vi "set_Mode.vi"(6 "Array":T1(array[cluster]), 7 "Array 3":string[](array[string]), 10 "Array 2":T1(array[cluster])) -> (2 "settings needed":bool, 3 "spreadsheet string":string)   [LabVIEW 2013, in "Tapedrive_ESP301.lvclass"]
uses:
  Tapedrive_ESP301.lvclass
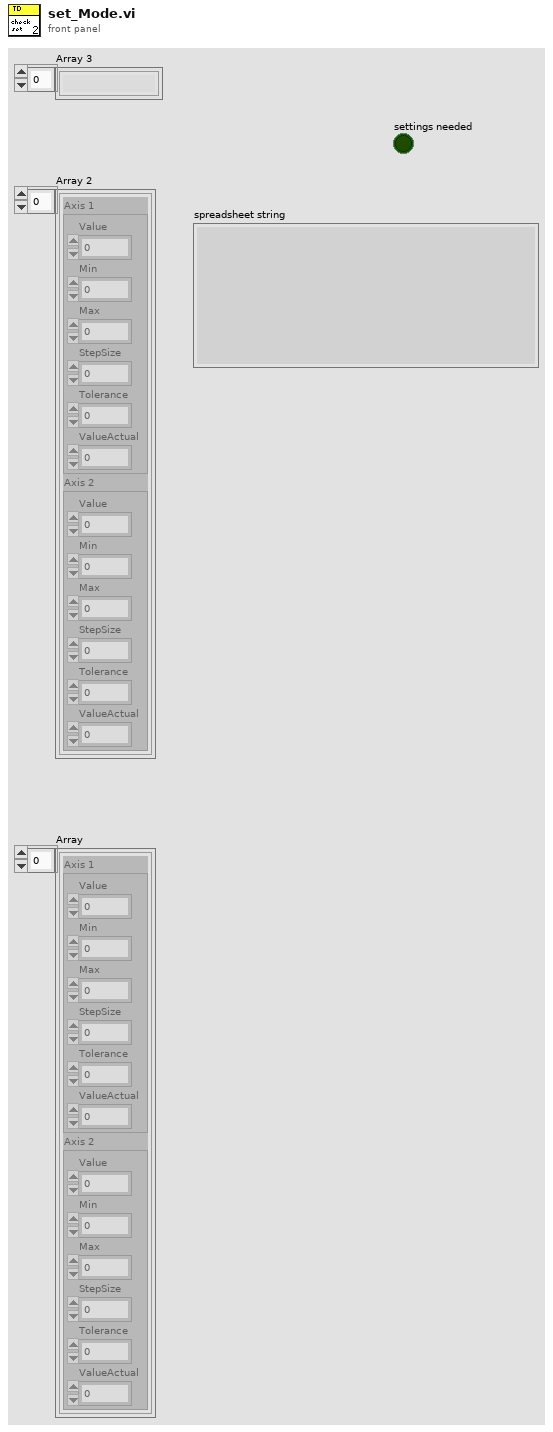
[diagram p1: front panel]
types:
  T1 = cluster{"Axis 1":cluster{"Value":dbl, "Min":dbl, "Max":dbl, "StepSize":dbl, "Tolerance":dbl, "ValueActual":dbl}, "Axis 2":cluster{"Value":dbl, "Min":dbl, "Max":dbl, "StepSize":dbl, "Tolerance":dbl, "ValueActual":dbl}}[]
  T2 = cluster{"Axis 1":cluster{"Value":bool, "Min":bool, "Max":bool, "StepSize":bool, "Tolerance":bool, "ValueActual":bool}, "Axis 2":cluster{"Value":bool, "Min":bool, "Max":bool, "StepSize":bool, "Tolerance":bool, "ValueActual":bool}}
  T3 = cluster{"Value":dbl, "Min":dbl, "Max":dbl, "StepSize":dbl, "Tolerance":dbl, "ValueActual":dbl}[]
  T4 = cluster{"Value":bool, "Min":bool, "Max":bool, "StepSize":bool, "Tolerance":bool, "ValueActual":bool}[]
  T5 = cluster{"Value":dbl, "Min":dbl, "Max":dbl, "StepSize":dbl, "Tolerance":dbl, "ValueActual":dbl}
  T6 = cluster{"Value":bool, "Min":bool, "Max":bool, "StepSize":bool, "Tolerance":bool, "ValueActual":bool}
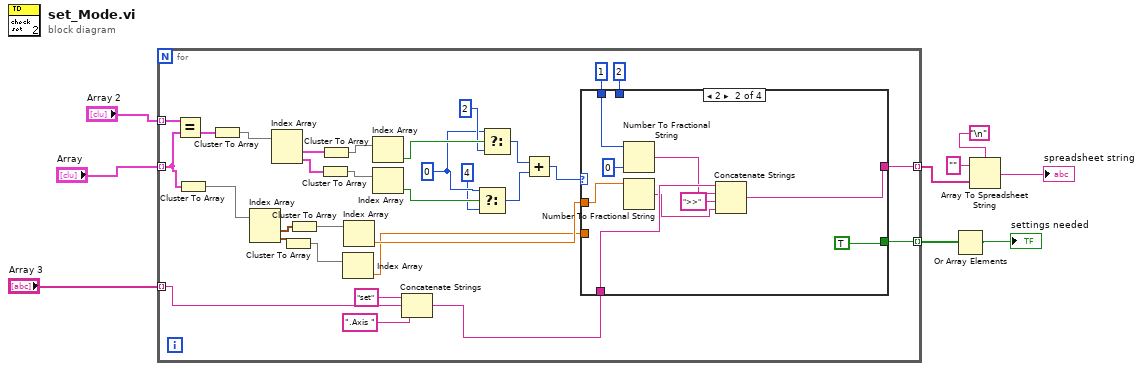
[diagram p0: block diagram]
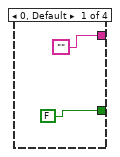
[diagram p2: hidden frame]
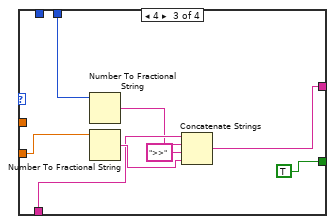
[diagram p3: hidden frame]
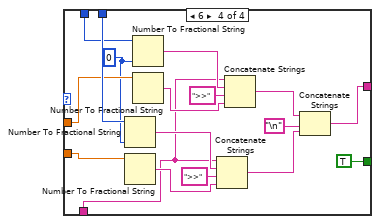
[diagram p4: hidden frame]
diagram:
  n1 = for {
    tunnel: "Array 3" -> [w19] mode=indexing
    tunnel: "Array 2" -> [w18] mode=indexing
    tunnel: "Array" -> [w17] mode=indexing
    tunnel: [w16] -> w9 mode=indexing
    tunnel: [w15] -> w2 mode=indexing
    w11 = 0
    n2 = Equal?(x=w18, y=w17) -> (x = y?=w40:T2)
    n3 = Cluster To Array(cluster=w17) -> (array=w32:T3)
    n4 = Cluster To Array(cluster=w40) -> (array=w39:T4)
    n5 = Index Array(array=w32) -> (element #1=w31:T5, element #2=w30:T5)  [unwired: 2 in]
    n6 = Index Array(array=w39) -> (element #1=w38:T6, element #2=w37:T6)  [unwired: 2 in]
    n7 = Cluster To Array(cluster=w30) -> (array=w28:dbl[])
    n8 = Cluster To Array(cluster=w31) -> (array=w29:dbl[])
    n9 = Cluster To Array(cluster=w37) -> (array=w35:bool[])
    n10 = Cluster To Array(cluster=w38) -> (array=w36:bool[])
    n11 = Index Array(array=w28) -> (element=w23:dbl)  [unwired: 1 in]
    n12 = Index Array(array=w29) -> (element=w24:dbl)  [unwired: 1 in]
    n13 = Index Array(array=w36) -> (element=w34:bool)  [unwired: 1 in]
    n14 = Index Array(array=w35) -> (element=w33:bool)  [unwired: 1 in]
    n15 = Concatenate Strings("set" ("string"), w19, ".Axis " ("string")) -> (w20:string)
    n16 = Select(t=w11, s=w33, f=4) -> (s? t:f=w26:i32)
    n17 = Select(t=w11, s=w34, f=2) -> (s? t:f=w27:i32)
    n18 = Add(x=w27, y=w26) -> (x+y=w25:i32)
    n19 = case shown="2" w25 {
      tunnel: w24 -> [_ w51 _ w66]
      tunnel: w23 -> [_ _ w57 w69]
      tunnel: w20 -> [_ w50 w55 w70]
      tunnel: i16 1 ("forwardaxis") -> [_ w49 _ w67]
      tunnel: i16 2 ("backwardaxis") -> [_ _ w56 w68]
      tunnel: ["" w45 w54 w62] -> w16
      tunnel: [FALSE TRUE TRUE TRUE] -> w15
      frame 0, Default {
      }
      frame 2 {
        n20 = Number To Fractional String(number=w49, precision (6)=i16 0) -> (F-format string=w48:string)  [unwired: 2 in]
        n21 = Number To Fractional String(number=w51) -> (F-format string=w46:string)  [unwired: 3 in]
        n22 = Concatenate Strings(w50, w48, ">>" ("string"), w46) -> (w45:string)
      }
      frame 4 {
        n23 = Number To Fractional String(number=w56) -> (F-format string=w52:string)  [unwired: 3 in]
        n24 = Number To Fractional String(number=w57) -> (F-format string=w58:string)  [unwired: 3 in]
        n25 = Concatenate Strings(w55, w52, ">>" ("string"), w58) -> (w54:string)
      }
      frame 6 {
        w60 = i16 0 ("width (-)")
        n26 = Number To Fractional String(number=w68, precision (6)=w60) -> (F-format string=w76:string)  [unwired: 2 in]
        n27 = Number To Fractional String(number=w69) -> (F-format string=w74:string)  [unwired: 3 in]
        n28 = Number To Fractional String(number=w67, precision (6)=w60) -> (F-format string=w71:string)  [unwired: 2 in]
        n29 = Number To Fractional String(number=w66) -> (F-format string=w73:string)  [unwired: 3 in]
        n30 = Concatenate Strings(w70, w76, ">>" ("string"), w74) -> (w64:string)
        n31 = Concatenate Strings(w70, w71, ">>" ("string"), w73) -> (w65:string)
        n32 = Concatenate Strings(w65, "\n", w64) -> (w62:string)
      }
    }
  }
  n33 = Or Array Elements(Boolean array=w2) -> (logical OR=→"settings needed":bool)
  n34 = Array To Spreadsheet String(delimiter (Tab)="\n", array=w9, 3:"" ("format string")) -> (spreadsheet string=→"spreadsheet string":string)
